vi "Write General Setting to PVM.vi"(11 "UI General Setting in":T1) -> (3 "UI General Setting out":T1)   [LabVIEW 2015, in "ConfigHelper.lvlib"]
uses:
  ConfigHelper.lvlib
  Control_UI_General Setting.ctl
  Control_UI_General Setting State.ctl
  <vilib>/addons/PointValueMap/controls/PointMap.ctl
  Control_General Setup (Path).ctl
  <vilib>/addons/PointValueMap/PointValueMap.lvlib
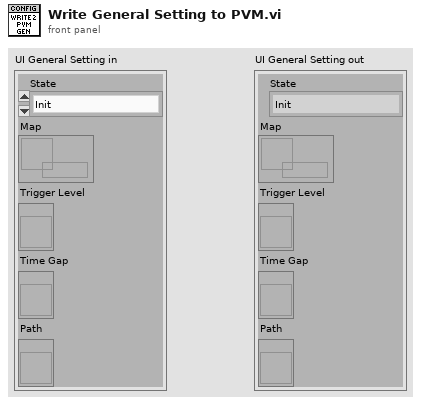
[diagram p1: front panel]
types:
  T1 = typedef "ConfigHelper.lvlib/Control_UI_General Setting.ctl" = cluster{"State":T2, "Map":T3, "Trigger Level":refnum<vi>, "Time Gap":refnum<vi>, "Path":refnum<vi>}
  T2 = typedef "ConfigHelper.lvlib/Control_UI_General Setting State.ctl" = enum16{"Init", "Wait", "Write to PVM", "Exit"}
  T3 = typedef "PointValueMap.lvlib/PointMap.ctl" = refnum<data-value>
  T4 = typedef "ConfigHelper.lvlib/Control_General Setup (Path).ctl" = cluster{"Export Path":path, "level":dbl, "Time Gap":dbl}
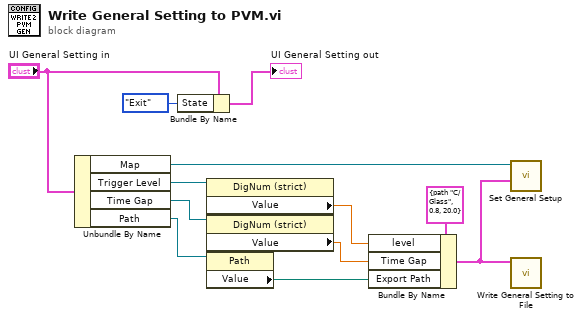
[diagram p0: block diagram]
diagram:
  n1 = Unbundle By Name("UI General Setting in") -> ("Map"=w6:T3, "Trigger Level"=w12:refnum<vi>, "Time Gap"=w11:refnum<vi>, "Path"=w10:refnum<vi>)
  n2 = Bundle By Name(cluster="UI General Setting in", "State"=Control_UI_General_Setting_State."Exit") -> (→"UI General Setting out":T1)
  n3 = property class="DigNum (strict)"(reference=w12) -> ("Value"=w7:dbl)  [unwired: 1 in, 2 out]
  n4 = property class="DigNum (strict)"(reference=w11) -> ("Value"=w8:dbl)  [unwired: 1 in, 2 out]
  n5 = property class="Path"(reference=w10) -> ("Value"=w1:path)  [unwired: 1 in, 2 out]
  n6 = Bundle By Name(cluster=T4 {"Export Path"=path "C:/Glass", "level"=0.8, "Time Gap"=20.0} ("General Setup"), "level"=w7, "Time Gap"=w8, "Export Path"=w1) -> (w2:T4)
  n7 = call "Set General Setup.vi"("General Setup"=w2, "Map"=w6) -> ()  [unwired: 8 in, 2 out]
  n8 = call "Write General Setting to File.vi"("General Setup"=w2) -> ()  [unwired: 11 in]
